vi "PruebaGit.vi"() -> ()   [LabVIEW 2020]
panel:
  out "before substring 3":string
  out "before substring 2":string
  out "after substring 2":string
  out "match substring":string
  out "after substring":string
  out "before substring":string
  out "date/time string":string
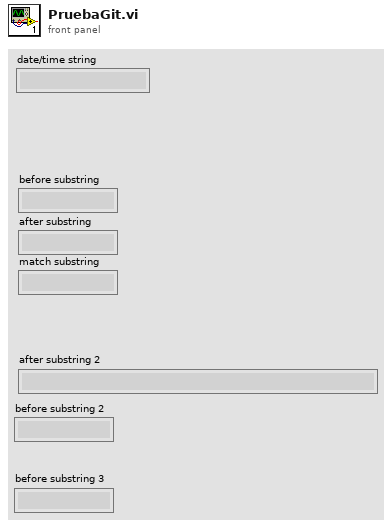
[diagram p1: front panel]
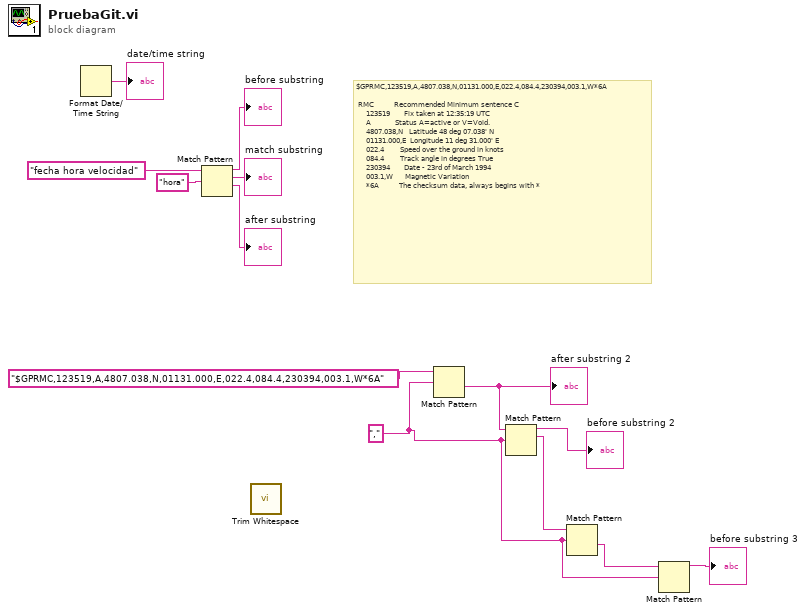
[diagram p0: block diagram]
diagram:
  w2 = "," ("regular expression")
  # "$GPRMC,123519,A,4807.038,N,01131.000,E,022.4,084.4,230394,003.1,W*6A\n\n RMC          Recommended Minimum sentence C\n     123519       Fix taken at 12:35:19 UTC\n     A            Status A=active or V=Void.\n     4807.038,N   Latitude 48 deg 07.038' N\n     01131.000,E  Longitude 11 deg 31.000' E\n     022.4        Speed over the ground in knots\n     084.4        Track angle in degrees True\n     230394       Date - 23rd of March 1994\n     003.1,W      Magnetic Variation\n     *6A          The checksum data, always begins with *"
  n1 = Format Date/Time String() -> (date/time string=→"date/time string":string)  [unwired: 3 in]
  n2 = Match Pattern(string="fecha hora velocidad", regular expression="hora") -> (before substring=→"before substring":string, match substring=→"match substring":string, after substring=→"after substring":string)  [unwired: 1 in, 1 out]
  n3 = call <vilib>:"Trim Whitespace.vi"() -> ()  [unwired: 2 in, 1 out]
  n4 = Match Pattern(string="$GPRMC,123519,A,4807.038,N,01131.000,E,022.4,084.4,230394,003.1,W*6A", regular expression=w2) -> (after substring=w6:string)  [unwired: 1 in, 3 out]
  "after substring 2" <- w6
  n5 = Match Pattern(string=w6, regular expression=w2) -> (before substring=→"before substring 2":string, match substring=w4:string)  [unwired: 1 in, 2 out]
  n6 = Match Pattern(string=w4, regular expression=w2) -> (after substring=w1:string)  [unwired: 1 in, 3 out]
  n7 = Match Pattern(string=w1, regular expression=w2) -> (before substring=→"before substring 3":string)  [unwired: 1 in, 3 out]
